vi "testChem3.vi"() -> ()   [LabVIEW 2012]
uses:
  <userlib>/ImageProcessing/InitCamera_NTSC.vi
  <vilib>/Utility/file.llb/Read From Spreadsheet File (string).vi
  <userlib>/ImageProcessing/FilterGreenPlane.vi
  <userlib>/ImageProcessing/FilterRedPlane.vi
panel:
  out "Array":string[](array[string])
  out "Element":string[](array[string])
  out "Min":dbl[](array[numeric])
  out "Max":dbl[](array[numeric])
  out "S4":dbl[](array[numeric])
  out "S3":dbl[](array[numeric])
  out "S2":dbl[](array[numeric])
  out "S1":dbl[](array[numeric])
  in  "Path":path
  out "Periodic":string[][](array[string])
  out "indexsWhereTrue":i32[](array[numeric])
  out "x+y":dbl[](array[numeric])
  out "image 2":picture
  out "Ra4":dbl
  out "Ra3":dbl
  out "Ra2":dbl
  out "Ra1":dbl
  out "A4":dbl
  out "A3":dbl
  out "A2":dbl
  out "A1":dbl
  out "a4":dbl
  out "a3":dbl
  out "a2":dbl
  out "a1":dbl
  out "Centroid 4":cluster{"X":dbl, "Y":dbl}
  out "Centroid 3":cluster{"X":dbl, "Y":dbl}
  out "Centroid 2":cluster{"X":dbl, "Y":dbl}
  out "Centroid":cluster{"X":dbl, "Y":dbl}
  out "initialized array 2":dbl[][](array[numeric])
  out "image":picture
  in  "Stop":bool
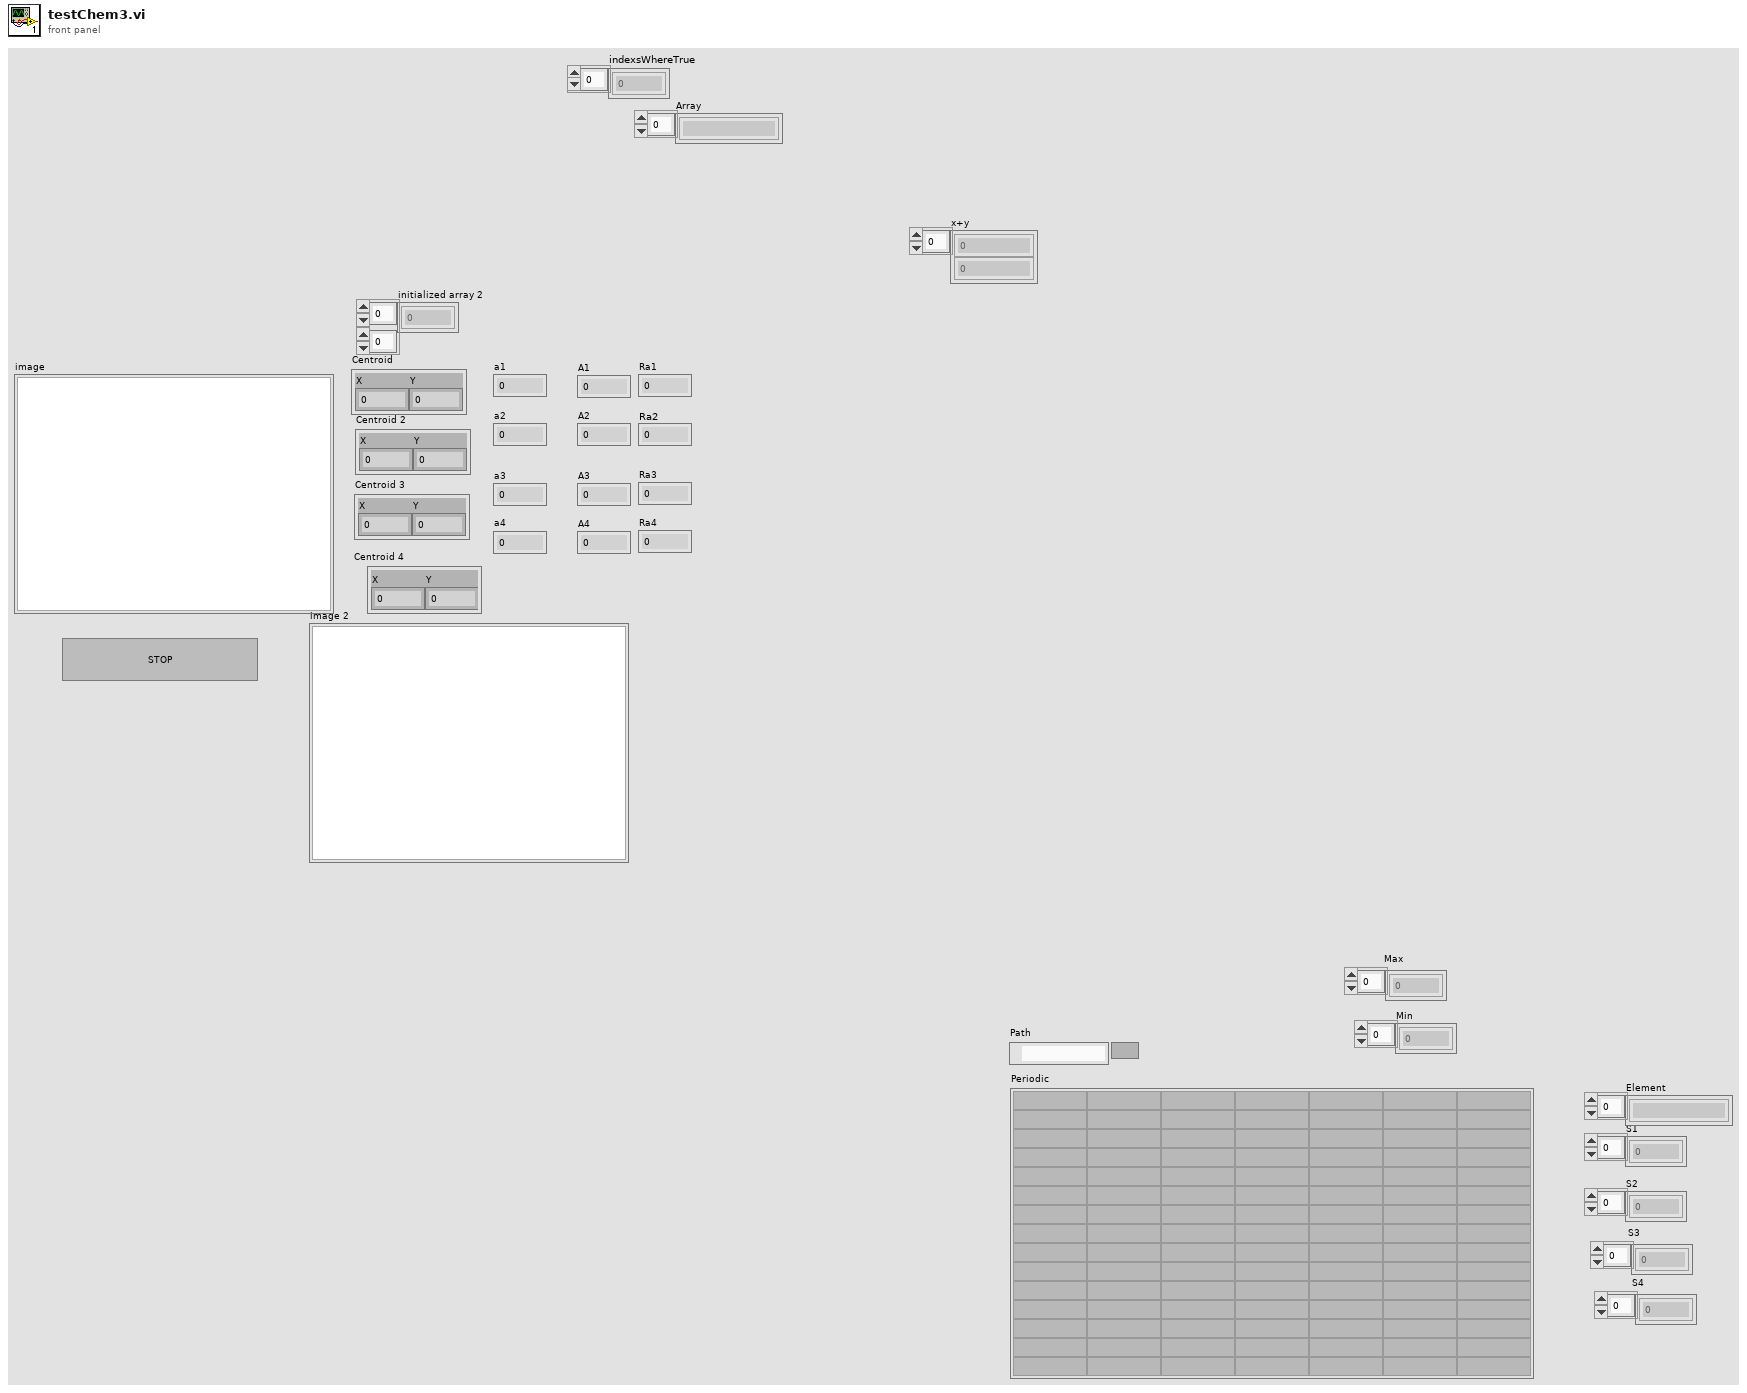
[diagram p1: front panel]
types:
  T1 = typedef "QT_Ref.ctl" = refnum<k1>
  T2 = cluster{"Width":u16, "Style":enum32{"Solid", "Dash", "Dot", "DashDot", "DashDotDot"}}
  T3 = typedef "QT_Image.ctl" = cluster{"Width":i32, "Height":i32, "Depth":i32, "data":u8[], "Compressed data":u8[], "Color table":u32[], "Duration":i32, "Options":i32, "Timestamp":i32, "ID":i32, "Reserved":i32, "Dialogs":u32}
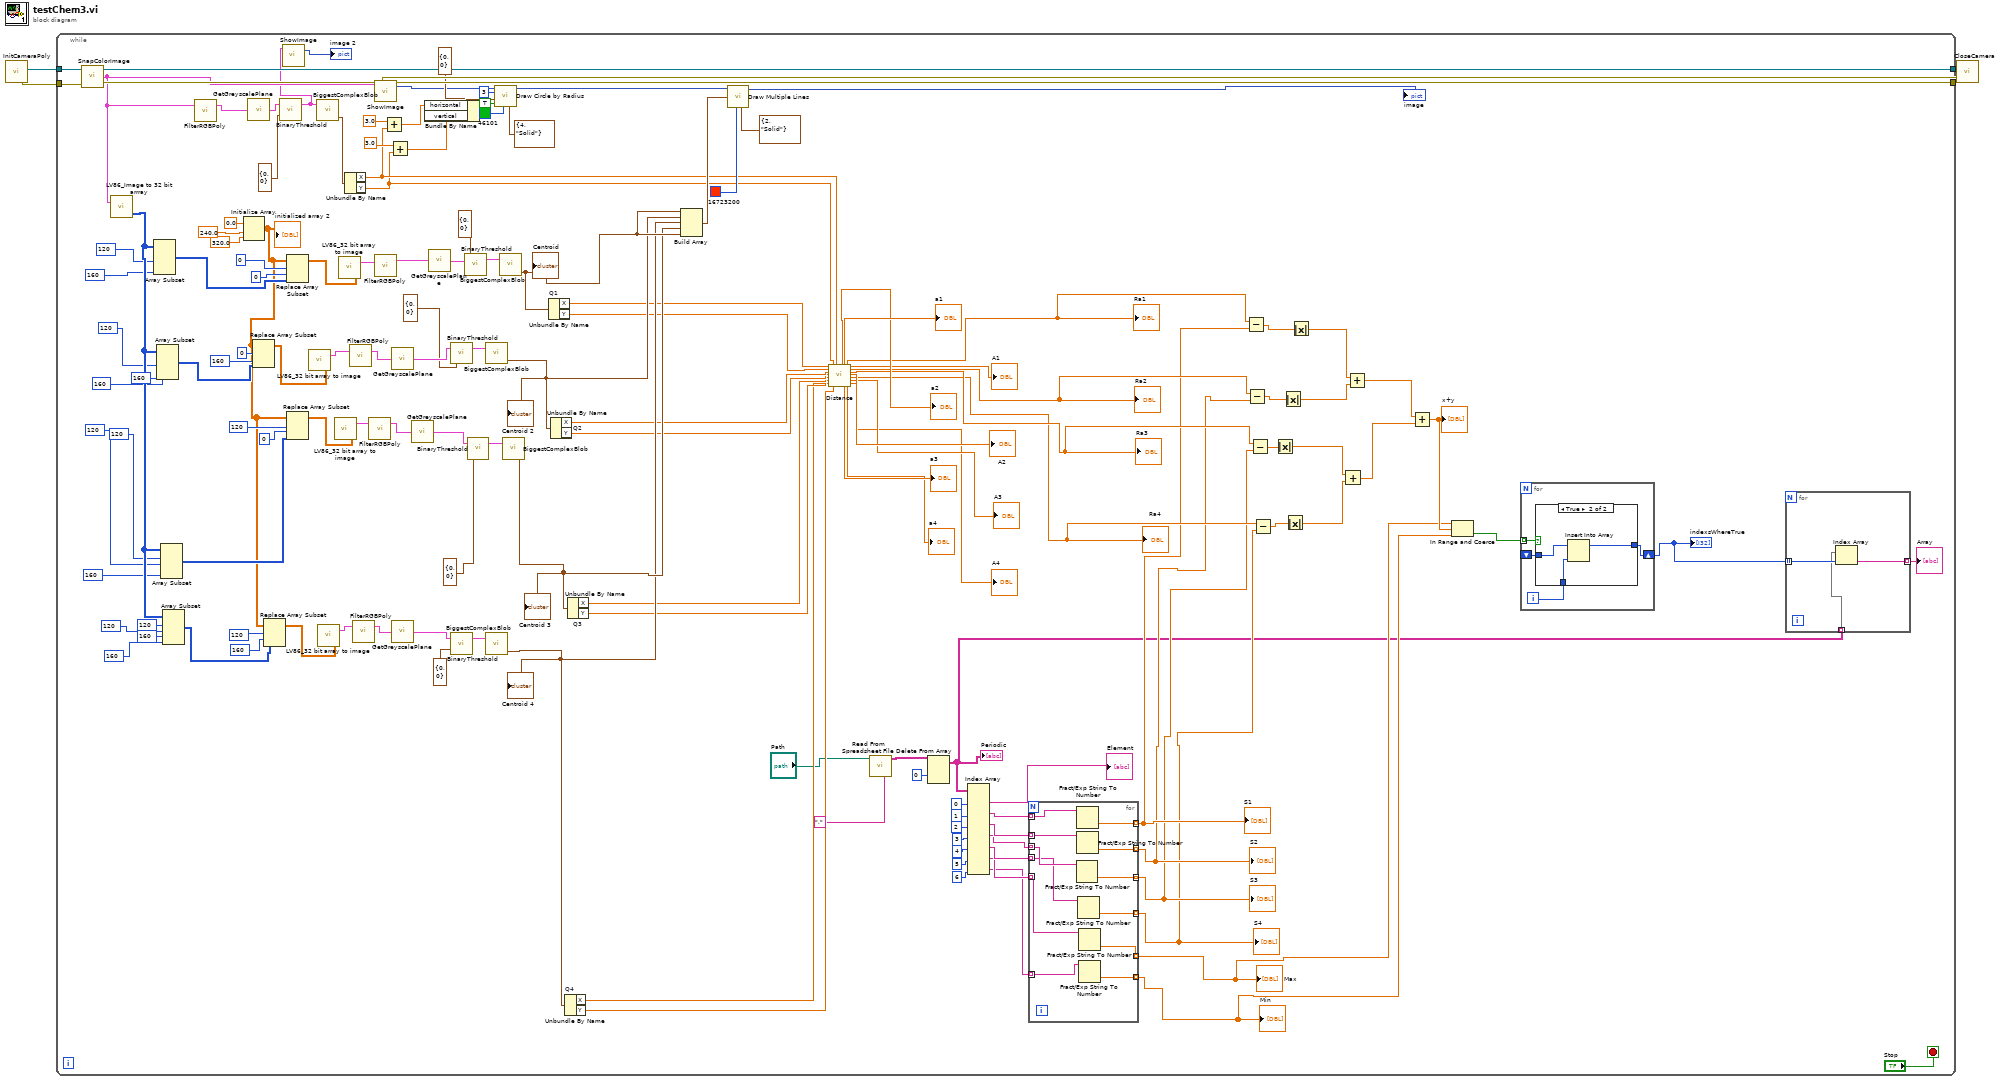
[diagram p0: block diagram]
diagram:
  n1 = call-poly <userlib>:"InitCameraPoly.vi"() -> ("error out"=w1:errorcluster, "QT Ref Out"=w2:T1)  [unwired: 2 in]
  n2 = while {
    tunnel: w1 -> [w150]
    tunnel: w2 -> [w149]
    tunnel: [w148] -> w3
    tunnel: [w147] -> w4
    stop <- "Stop" stop-if-true
    n3 = call <userlib>:"SnapColorImage.vi"("error in (no error)"=w150, "QT Ref In"=w149) -> ("error out"=w148:errorcluster, "Image Out"=w81:T3, "QT Ref Out"=w147:T1)  [unwired: 1 in]
    n4 = call <userlib>:"LV86_Image to 32 bit arrray.vi"("Image In"=w81) -> ("Intensity Graph"=w145:u32[][])  [unwired: 1 in, 1 out]
    n5 = Array Subset(array=w145, length (row)=120 ("length"), length (col)=160 ("length")) -> (w121:u32[][])  [unwired: 2 in]
    n6 = Array Subset(array=w145, length (row)=120 ("length"), index (col)=160 ("index"), length (col)=160 ("length")) -> (w132:u32[][])  [unwired: 1 in]
    n7 = Array Subset(array=w145, index (row)=120 ("index"), length (row)=120 ("length"), length (col)=160 ("length")) -> (w115:u32[][])  [unwired: 1 in]
    n8 = Array Subset(array=w145, index (row)=120 ("index"), length (row)=120 ("length"), index (col)=160 ("index"), length (col)=160 ("length")) -> (w112:u32[][])
    n9 = call-poly <userlib>:"FilterRGBPoly.vi"("Image in"=w81) -> ("Image out"=w84:T3)  [unwired: 1 in, 1 out]
    n10 = Initialize Array(0.0 ("element"), 240.0 ("element"), 320.0 ("element")) -> (w111:dbl[][])
    "initialized array 2" <- w111
    n11 = call <userlib>:"GetGreyscalePlane.vi"("Image In"=w84) -> ("Greyscale  Out"=w68:T3)
    n12 = Replace Array Subset(array=w111, new element=w132, index (row)=0, index (col)=160 ("index (row)")) -> (w131:dbl[][])
    n13 = Replace Array Subset(array=w111, new element=w112, index (row)=120, index (col)=160 ("index (row)")) -> (w109:dbl[][])
    n14 = call <userlib>:"BinaryThreshold.vi"("threshold"=cluster{u8, u8} {0, 0}, "Image In"=w68) -> ("Image Out"=w66:T3)  [unwired: 1 in]
    n15 = call <userlib>:"ShowImage.vi"("Image"=w66) -> ("image"=→"image 2":picture)  [unwired: 2 in, 1 out]
    n16 = Replace Array Subset(array=w111, new element=w121, index (row)=0, index (col)=0 ("index (row)")) -> (w120:dbl[][])
    n17 = Replace Array Subset(array=w111, new element=w115, index (row)=120, index (col)=0 ("index (row)")) -> (w110:dbl[][])
    n18 = call <userlib>:"LV86_32 bit array to image.vi"("Intensity Graph"=w131) -> ("Image Out"=w108:T3)  [unwired: 2 in]
    n19 = call <userlib>:"BiggestComplexBlob.vi"("Image in"=w66) -> ("Centroid"=w82:cluster{"X":dbl, "Y":dbl})  [unwired: 1 in, 2 out]
    n20 = call <userlib>:"LV86_32 bit array to image.vi"("Intensity Graph"=w109) -> ("Image Out"=w106:T3)  [unwired: 2 in]
    n21 = call <userlib>:"LV86_32 bit array to image.vi"("Intensity Graph"=w110) -> ("Image Out"=w107:T3)  [unwired: 2 in]
    n22 = call <userlib>:"LV86_32 bit array to image.vi"("Intensity Graph"=w120) -> ("Image Out"=w119:T3)  [unwired: 2 in]
    n23 = Unbundle By Name(w82) -> ("X"=w65:dbl, "Y"=w64:dbl)
    n24 = call-poly <userlib>:"FilterRGBPoly.vi"("Image in"=w108) -> ("Image out"=w105:T3)  [unwired: 1 in, 1 out]
    n25 = call-poly <userlib>:"FilterRGBPoly.vi"("Image in"=w106) -> ("Image out"=w103:T3)  [unwired: 1 in, 1 out]
    n26 = call-poly <userlib>:"FilterRGBPoly.vi"("Image in"=w107) -> ("Image out"=w104:T3)  [unwired: 1 in, 1 out]
    n27 = call <userlib>:"ShowImage.vi"("Image"=w81) -> ("image"=w69:picture)  [unwired: 2 in, 1 out]
    n28 = call-poly <userlib>:"FilterRGBPoly.vi"("Image in"=w119) -> ("Image out"=w118:T3)  [unwired: 1 in, 1 out]
    n29 = Add(x=3.0, y=w65) -> (x+y=w75:dbl)
    n30 = Add(x=3.0, y=w64) -> (x+y=w74:dbl)
    n31 = call <userlib>:"GetGreyscalePlane.vi"("Image In"=w103) -> ("Greyscale  Out"=w97:T3)
    n32 = call <userlib>:"GetGreyscalePlane.vi"("Image In"=w105) -> ("Greyscale  Out"=w99:T3)
    n33 = call <userlib>:"GetGreyscalePlane.vi"("Image In"=w104) -> ("Greyscale  Out"=w98:T3)
    n34 = Bundle By Name(cluster=cluster{"horizontal":i16, "vertical":i16} {"horizontal"=0, "vertical"=0} ("pixel center"), "horizontal"=w75, "vertical"=w74) -> (w79:cluster{"horizontal":i16, "vertical":i16})
    n35 = call <userlib>:"GetGreyscalePlane.vi"("Image In"=w118) -> ("Greyscale  Out"=w117:T3)
    n36 = call <userlib>:"BinaryThreshold.vi"("threshold"=cluster{u8, u8} {0, 0}, "Image In"=w99) -> ("Image Out"=w102:T3)  [unwired: 1 in]
    n37 = call <userlib>:"BinaryThreshold.vi"("threshold"=cluster{u8, u8} {0, 0}, "Image In"=w97) -> ("Image Out"=w100:T3)  [unwired: 1 in]
    n38 = call <userlib>:"BinaryThreshold.vi"("threshold"=cluster{u8, u8} {0, 0}, "Image In"=w117) -> ("Image Out"=w116:T3)  [unwired: 1 in]
    n39 = call <userlib>:"BinaryThreshold.vi"("threshold"=cluster{u8, u8} {0, 0}, "Image In"=w98) -> ("Image Out"=w101:T3)  [unwired: 1 in]
    n40 = call <userlib>:"BiggestComplexBlob.vi"("Image in"=w102) -> ("Centroid"=w87:cluster{"X":dbl, "Y":dbl})  [unwired: 1 in, 2 out]
    "Centroid 2" <- w87
    n41 = call <userlib>:"BiggestComplexBlob.vi"("Image in"=w100) -> ("Centroid"=w85:cluster{"X":dbl, "Y":dbl})  [unwired: 1 in, 2 out]
    "Centroid 4" <- w85
    n42 = call <vilib>:"Draw Circle by Radius.vi"("pen"=T2 {"Width"=4, "Style"=enum."Solid"}, "color(black)"=u32 46101, "fill?(F)"=TRUE, "pixel center"=w79, "radius"=i16 3, "picture"=w69) -> ("new picture"=w80:picture)  [unwired: 5 in]
    n43 = call <userlib>:"BiggestComplexBlob.vi"("Image in"=w116) -> ("Centroid"=w88:cluster{"X":dbl, "Y":dbl})  [unwired: 1 in, 2 out]
    "Centroid" <- w88
    n44 = call <userlib>:"BiggestComplexBlob.vi"("Image in"=w101) -> ("Centroid"=w86:cluster{"X":dbl, "Y":dbl})  [unwired: 1 in, 2 out]
    "Centroid 3" <- w86
    n45 = Unbundle By Name "Q1"(w88) -> ("X"=w63:dbl, "Y"=w62:dbl)
    n46 = Unbundle By Name "Q2"(w87) -> ("X"=w61:dbl, "Y"=w60:dbl)
    n47 = Unbundle By Name "Q4"(w85) -> ("X"=w57:dbl, "Y"=w56:dbl)
    n48 = Unbundle By Name "Q3"(w86) -> ("X"=w59:dbl, "Y"=w58:dbl)
    n49 = Build Array(w88, w87, w85, w86, w88) -> (w95:cluster{"X":dbl, "Y":dbl}[])
    n50 = call <vilib>:"Draw Multiple Lines.vi"("picture"=w80, "line endpoints"=w95, "color(black)"=u32 16723200, "pen"=T2 {"Width"=2, "Style"=enum."Solid"}) -> ("new picture"=→"image":picture)  [unwired: 5 in]
    n51 = call "Distance.vi"("X1"=w63, "Y1"=w62, "X2"=w61, "Y2"=w60, "X3"=w59, "Y3"=w58, "x4"=w57, "Y"=w64, "Y4"=w56, "X"=w65) -> ("a2"=→"a2":dbl, "a1"=→"a1":dbl, "a3"=→"a3":dbl, "Ra1"=w47:dbl, "a4"=→"a4":dbl, "A1"=→"A1":dbl, "Ra2"=w46:dbl, "Ra3"=w45:dbl, "A2"=→"A2":dbl, "Ra4"=w44:dbl, "A3"=→"A3":dbl, "A4"=→"A4":dbl)  [unwired: 6 in]
    "Ra1" <- w47
    "Ra2" <- w46
    "Ra3" <- w45
    "Ra4" <- w44
    n52 = call-poly <vilib>:"Read From Spreadsheet File.vi"("delimiter (\\t)"="," ("delimiter (\\t)"), "file path (dialog if empty)"="Path") -> ("all rows"=w30:string[][])  [unwired: 5 in, 4 out]
    n53 = Delete From Array(array=w30, index (row)=0) -> (array with subset deleted=w6:string[][])  [unwired: 2 in, 1 out]
    "Periodic" <- w6
    n54 = Index Array(array=w6, index (col) #1=0 ("disabled index (col)"), index (col) #2=1 ("index (col)"), index (col) #3=2 ("index (col)"), index (col) #4=3 ("index (col)"), index (col) #5=4 ("index (col)"), index (col) #6=5 ("index (col)"), index (col) #7=6 ("index (col)")) -> (element #1=→"Element":string[], element #2=w23:string[], element #3=w22:string[], element #4=w19:string[], element #5=w18:string[], element #6=w15:string[], element #7=w14:string[])  [unwired: 7 in]
    n55 = for {
      tunnel: w23 -> [w162] mode=indexing
      tunnel: w22 -> [w161] mode=indexing
      tunnel: [w160] -> w13 mode=indexing
      tunnel: [w159] -> w12 mode=indexing
      tunnel: [w158] -> w11 mode=indexing
      tunnel: w19 -> [w157] mode=indexing
      tunnel: w18 -> [w156] mode=indexing
      tunnel: [w155] -> w10 mode=indexing
      tunnel: w15 -> [w154] mode=indexing
      tunnel: w14 -> [w153] mode=indexing
      tunnel: [w152] -> w9 mode=indexing
      tunnel: [w151] -> w8 mode=indexing
      n56 = Fract/Exp String To Number(string=w157) -> (number=w158:dbl)  [unwired: 3 in, 1 out]
      n57 = Fract/Exp String To Number(string=w162) -> (number=w160:dbl)  [unwired: 3 in, 1 out]
      n58 = Fract/Exp String To Number(string=w161) -> (number=w159:dbl)  [unwired: 3 in, 1 out]
      n59 = Fract/Exp String To Number(string=w156) -> (number=w155:dbl)  [unwired: 3 in, 1 out]
      n60 = Fract/Exp String To Number(string=w154) -> (number=w152:dbl)  [unwired: 3 in, 1 out]
      n61 = Fract/Exp String To Number(string=w153) -> (number=w151:dbl)  [unwired: 3 in, 1 out]
    }
    "S1" <- w13
    "S2" <- w12
    "S3" <- w11
    "S4" <- w10
    "Max" <- w9
    "Min" <- w8
    n62 = Subtract(x=w47, y=w13) -> (x-y=w43:dbl[])
    n63 = Subtract(x=w46, y=w12) -> (x-y=w42:dbl[])
    n64 = Subtract(x=w45, y=w11) -> (x-y=w41:dbl[])
    n65 = Subtract(x=w44, y=w10) -> (x-y=w40:dbl[])
    n66 = Absolute Value(x=w41) -> (abs(x)=w37:dbl[])
    n67 = Absolute Value(x=w42) -> (abs(x)=w38:dbl[])
    n68 = Absolute Value(x=w40) -> (abs(x)=w36:dbl[])
    n69 = Absolute Value(x=w43) -> (abs(x)=w39:dbl[])
    n70 = Add(x=w37, y=w36) -> (x+y=w34:dbl[])
    n71 = Add(x=w39, y=w38) -> (x+y=w35:dbl[])
    n72 = Add(x=w35, y=w34) -> (x+y=w32:dbl[])
    "x+y" <- w32
    n73 = In Range and Coerce(upper limit=w9, x=w32, lower limit=w8) -> (In Range?=w33:bool[])  [unwired: 1 out]
    n74 = for {
      tunnel: w33 -> [w169] mode=indexing
      shift-right: [w167] -> w31
      shift-left: _ -> [w166]
      i -> [w168]
      n75 = case shown="True" w169 {
        tunnel: w168 -> [_ w171]
        tunnel: [w170 w173] -> w167
        tunnel: w166 -> [w170 w172]
        frame False {
        }
        frame True {
          n76 = Insert Into Array(array=w172, new element=w171) -> (w173:i32[])  [unwired: 1 in]
        }
      }
    }
    "indexsWhereTrue" <- w31
    n77 = for {
      tunnel: w31 -> [w165] mode=indexing
      tunnel: w6 -> [w164] mode=indexing
      tunnel: [w163] -> w5 mode=indexing
      n78 = Index Array(array=w164, index=w165) -> (element=w163:string)
    }
    "Array" <- w5
  }
  n79 = call <userlib>:"CloseCamera.vi"("error in (no error)"=w3, "QT Ref In"=w4) -> ()  [unwired: 1 in, 1 out]
